vi "MessageRobot.vi"(8 "Enemy Robots?":bool, 11 "Robot":T1={"id"=0, "function"=enum."Attacker", "x"=0.0, "y"=0.0, "orientation"=0.0, "v_tangent"=0.0, "v_normal"=0.0, "v_ang"=0.0, "kick_x"=0.0, "kick_z"=0.0, "dribble"=FALSE, "Timestamp"=timestamp(0 s since 1904-01-01), "estimatives"={"est_v_tangent"=0.0, "est_v_normal"=0.0, "est_vx"=0.0, "est_vy"=0.0, "Pos Robot Est"=[]}, "dest_x_kick"=0.0, "dest_y_kick"=0.0, "Gap Coord"=[], "States"=enum."GoToTangent", "Path "=[], "Path  Smooth"=[], "Dest"=[], "vx_desired"=0.0, "vy_desired"=0.0, "slowBehavior"=FALSE, "VSSStates"=enum."Pass"}) -> (1 "Array":u8[](array[numeric]))   [LabVIEW 2023]
uses:
  Vision_class/Old vision/Controls/AI Robot.ctl
  Vision_class/Old vision/Controls/Functions Enum.ctl
  Vision_class/Old vision/Controls/AttackerStates.ctl
  Vision_class/Old vision/Controls/PathDests.ctl
  Vision_class/Old vision/Controls/PathDest.ctl
  Game_class/Navigation/VSSNavigation/VSSAttackerStates.ctl
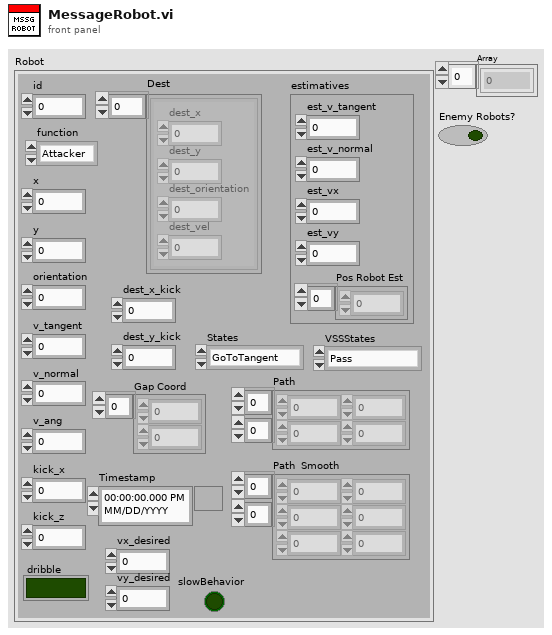
[diagram p1: front panel]
types:
  T1 = typedef "AI Robot.ctl" = cluster{"id":u32, "function":T2, "x":dbl, "y":dbl, "orientation":dbl, "v_tangent":dbl, "v_normal":dbl, "v_ang":dbl, "kick_x":dbl, "kick_z":dbl, "dribble":bool, "Timestamp":timestamp, "estimatives":cluster{"est_v_tangent":dbl, "est_v_normal":dbl, "est_vx":dbl, "est_vy":dbl, "Pos Robot Est":dbl[]}, "dest_x_kick":dbl, "dest_y_kick":dbl, "Gap Coord":dbl[], "States":T3, "Path ":dbl[][], "Path  Smooth":dbl[][], "Dest":T4, "vx_desired":dbl, "vy_desired":dbl, "slowBehavior":bool, "VSSStates":T6}
  T2 = typedef "Functions Enum.ctl" = enum16{"2nd Striker", "Attacker", "Goalie", "Defender", "Striker", "Goto 0", "Dummy", "Kicker", "ZigZag 0", "ZigZag 1", "ZigZag 2", "ZigZag 3", "ZigZag 4", "ZigZag 5", "ZigZag 6", "ZigZag 7", "ZigZag 8", ""}
  T3 = typedef "AttackerStates.ctl" = enum16{"Pass", "GoToTangent", "BallGetting", "GoToKick", ""}
  T4 = typedef "PathDests.ctl" = T5[]
  T5 = typedef "PathDest.ctl" = cluster{"dest_x":dbl, "dest_y":dbl, "dest_orientation":dbl, "dest_vel":dbl}
  T6 = typedef "VSSAttackerStates.ctl" = enum16{"Pass", "GoToTangent", "BallGetting", "GoToKick", "Rotate anti-clockwise", "Rotate Clockwise", ""}
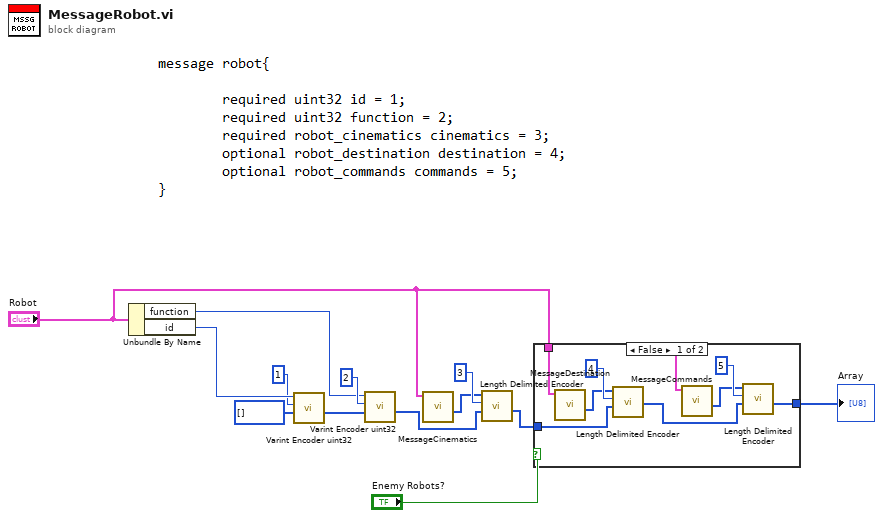
[diagram p0: block diagram]
diagram:
  n1 = Unbundle By Name("Robot") -> ("function"=w9:T2, "id"=w13:u32)
  n2 = call "Varint Encoder uint32.vi"("Array In"=u8[] [], "Key"=u32 1, "Value"=w13) -> ("Array"=w11:u8[])  [unwired: 8 in]
  n3 = call "Varint Encoder uint32.vi"("Array In"=w11, "Key"=u32 2, "Value"=w9) -> ("Array"=w7:u8[])  [unwired: 8 in]
  n4 = call "MessageCinematics.vi"("Robot"="Robot") -> ("Array"=w5:u8[])  [unwired: 10 in]
  n5 = call "Length Delimited Encoder.vi"("Array In"=w7, "Key"=u32 3, "Array In 2"=w5) -> ("Array"=w6:u8[])  [unwired: 8 in]
  n6 = case shown="False" "Enemy Robots?" {
    tunnel: w6 -> [w19 w22]
    tunnel: "Robot" -> [w15 _]
    tunnel: [w14 w22] -> w3
    frame False {
      n7 = call "MessageDestination.vi"("Robot"=w15) -> ("Array"=w20:u8[])  [unwired: 10 in]
      n8 = call "Length Delimited Encoder.vi"("Array In"=w19, "Key"=u32 4, "Array In 2"=w20) -> ("Array"=w16:u8[])  [unwired: 8 in]
      n9 = call "MessageCommands.vi"("Robot"=w15) -> ("Array"=w17:u8[])  [unwired: 10 in]
      n10 = call "Length Delimited Encoder.vi"("Array In"=w16, "Key"=u32 5, "Array In 2"=w17) -> ("Array"=w14:u8[])  [unwired: 8 in]
    }
    frame True {
    }
  }
  "Array" <- w3
